vi "FGV_DOCK_records_display.vi"(7 "options":T1, 8 "error_in":errorcluster, 11 "input":variant) -> (0 "error_out":errorcluster, 3 "output":variant)   [LabVIEW 2019]
uses:
  FGV_DOCK_records_display.ctl
  DOCK_references.ctl
  DOCK_all_info.ctl
  DOCK_reference_data.ctl
  MAIN/DOCK_header_data_display.ctl
  DOCK_gear_statuses.ctl
  _misc/AULocalize/SubVIs/Get Localized Phrase Compact Interface 0D.vi
  _misc/AULocalize/SubVIs/Get Localized Phrase Compact Interface 1D.vi
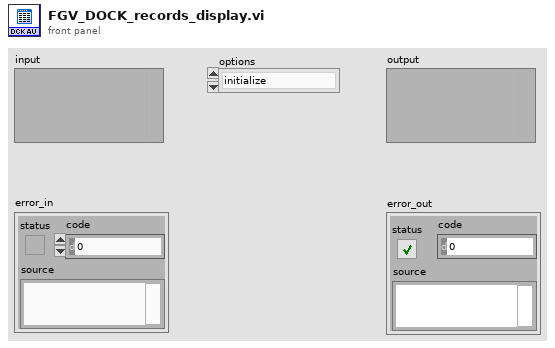
[diagram p1: front panel]
types:
  T1 = typedef "FGV_DOCK_records_display.ctl" = enum16{"initialize", "set_reference_data", "set_serial", "set_header", "set_operations", "set_results", "set_batches", "get_reference_data", "get_part_number_ref", "get_serial", "get_batch_code", "get_gear_ID", "get_operation_IDs", "toggle_results", "show_all_results", "hide_all_results", "display", "clear"}
  T2 = typedef "DOCK_all_info.ctl" = cluster{"reference_data":T3, "serial":string, "DOCK_header":T4, "operations":string[][], "operation_statuses":T5[], "results":string[][], "result_statuses":T5[], "batches":string[][], "batch_statuses":T5[], "DOCK_references":T6}
  T3 = typedef "DOCK_reference_data.ctl" = cluster{"part_number_ref":string, "part_name_ref":string, "PSW_ref":string, "AUSS_ref":string}
  T4 = typedef "DOCK_header_data_display.ctl" = cluster{"ID":string, "creation_time":string, "last_station":string, "last_status":string, "pinion_serial":string, "batch_code":string}
  T5 = typedef "DOCK_GEAR_statuses.ctl" = enum16{"OP_OK_hide", "OP_OK_show", "OP_NOK_hide", "OP_NOK_show", "OP_interrupted_hide", "OP_interrupted_show", "OP_in_operation_hide", "OP_in_operation_show", "OP_unexpected_hide", "OP_unexpected_show", "RE_REAL_OK", "RE_REAL_NOK", "RE_STRING", "RE_sub_header", "RE_no_data", "RE_unexpected", "BA_sub_header", "BA_data", "BA_no_data"}
  T6 = typedef "DOCK_references.ctl" = cluster{"front_panel_reference":refnum<vi>, "SQL_listbox_reference":refnum<vi>, "DOCK_header_data_display":refnum<vi>}
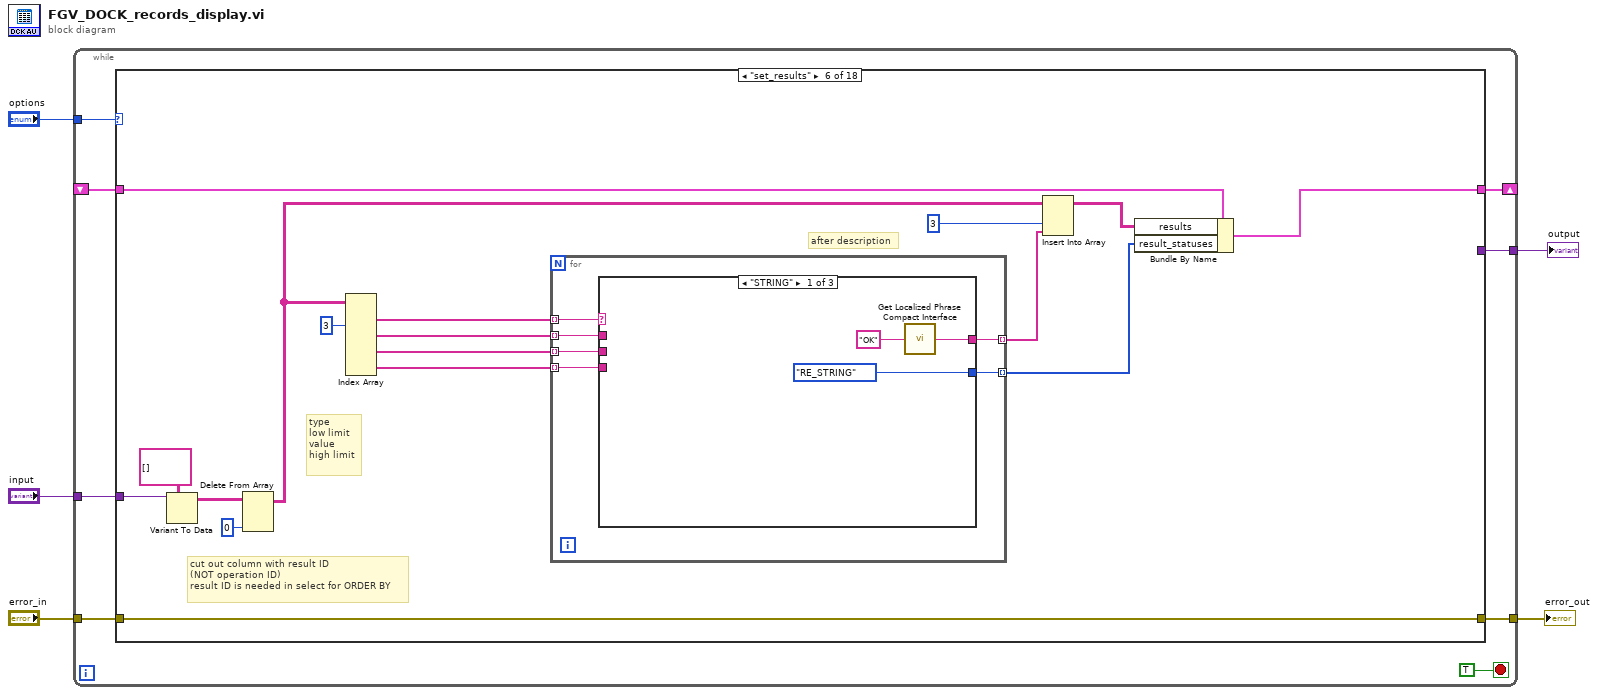
[diagram p0: block diagram]
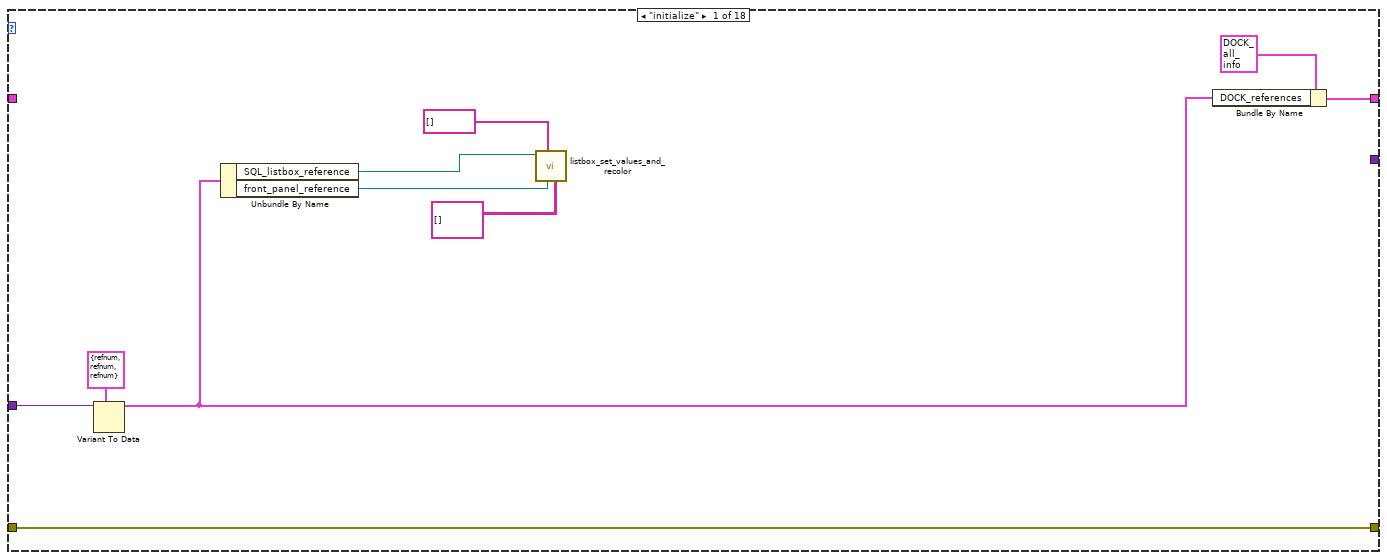
[diagram p2: hidden frame]
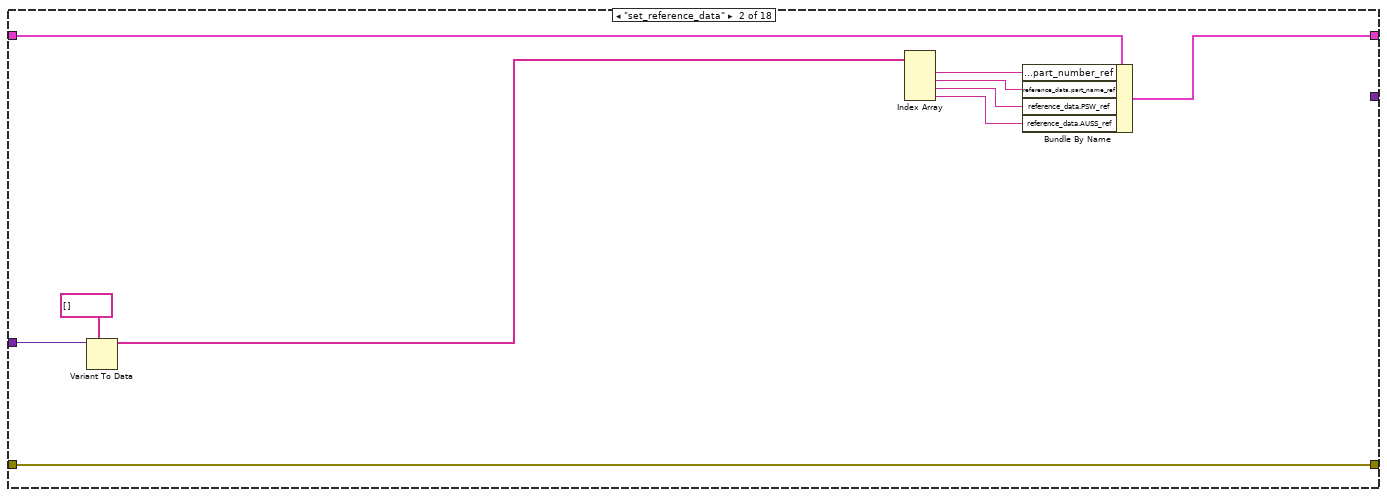
[diagram p3: hidden frame]
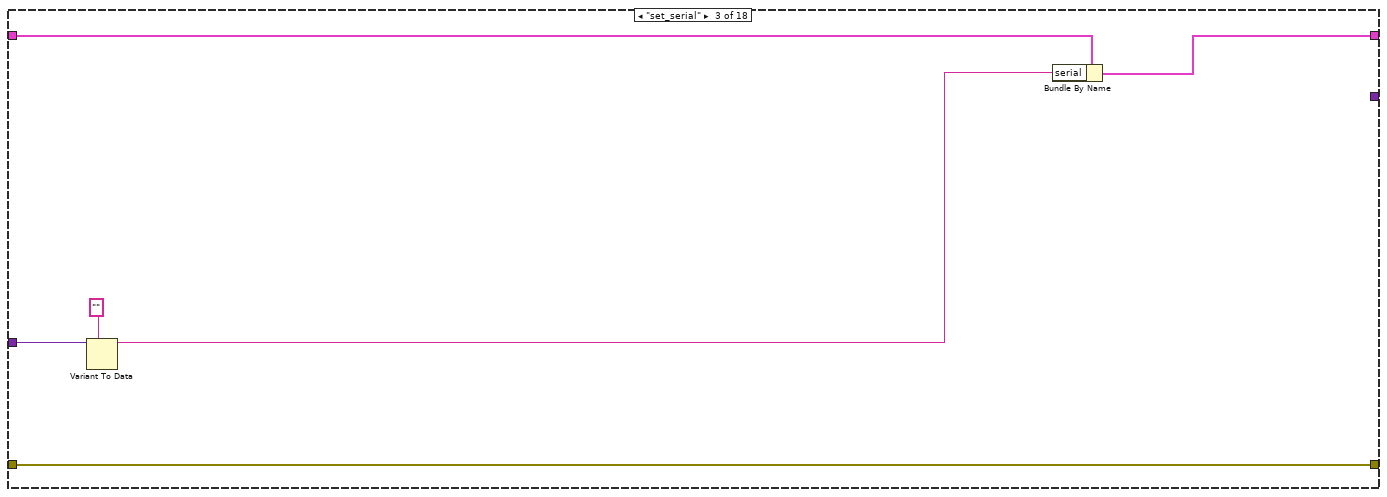
[diagram p4: hidden frame]
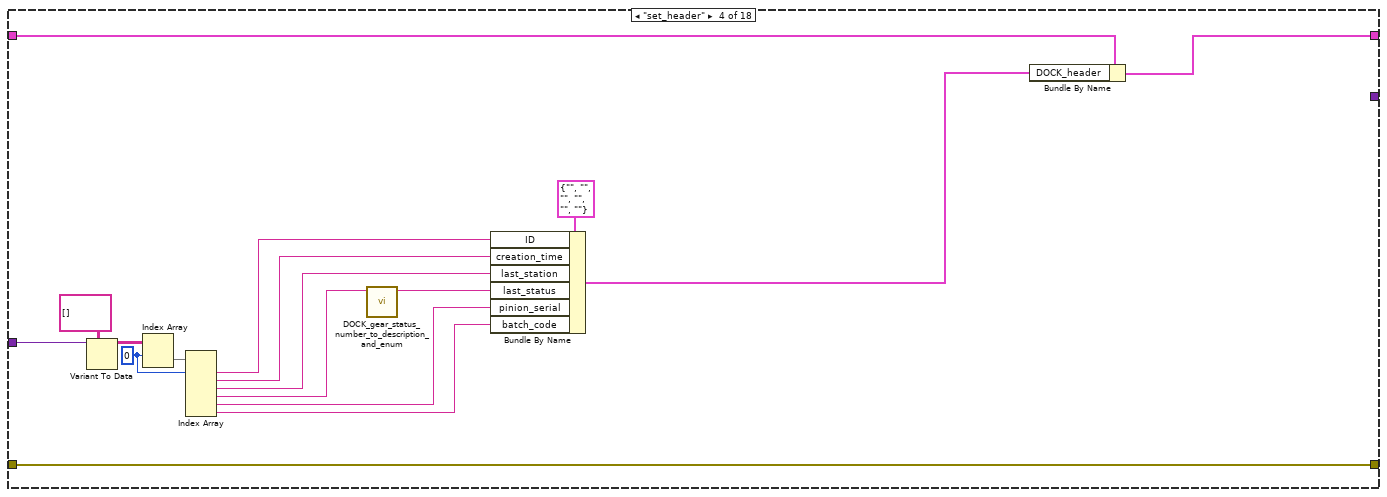
[diagram p5: hidden frame]
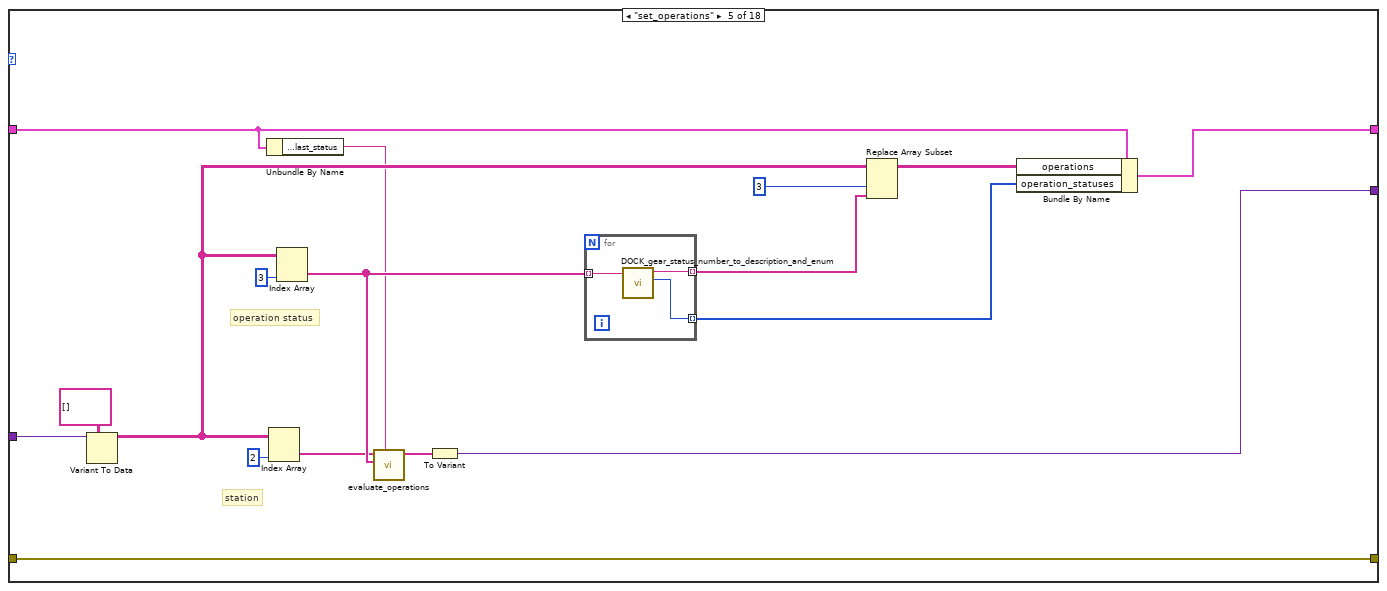
[diagram p6: hidden frame]
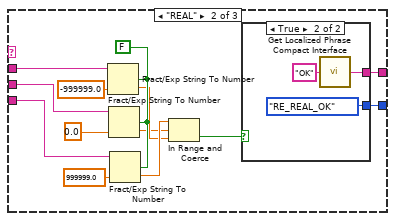
[diagram p7: hidden frame]
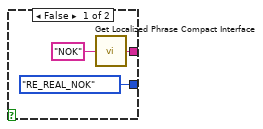
[diagram p8: hidden frame]
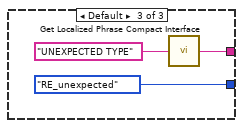
[diagram p9: hidden frame]
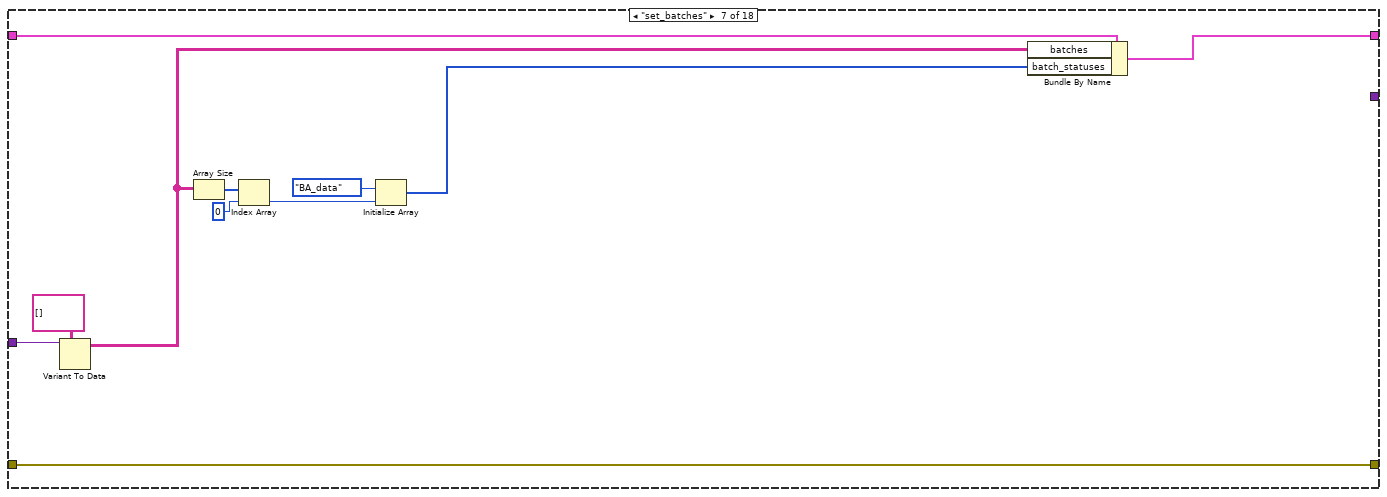
[diagram p10: hidden frame]
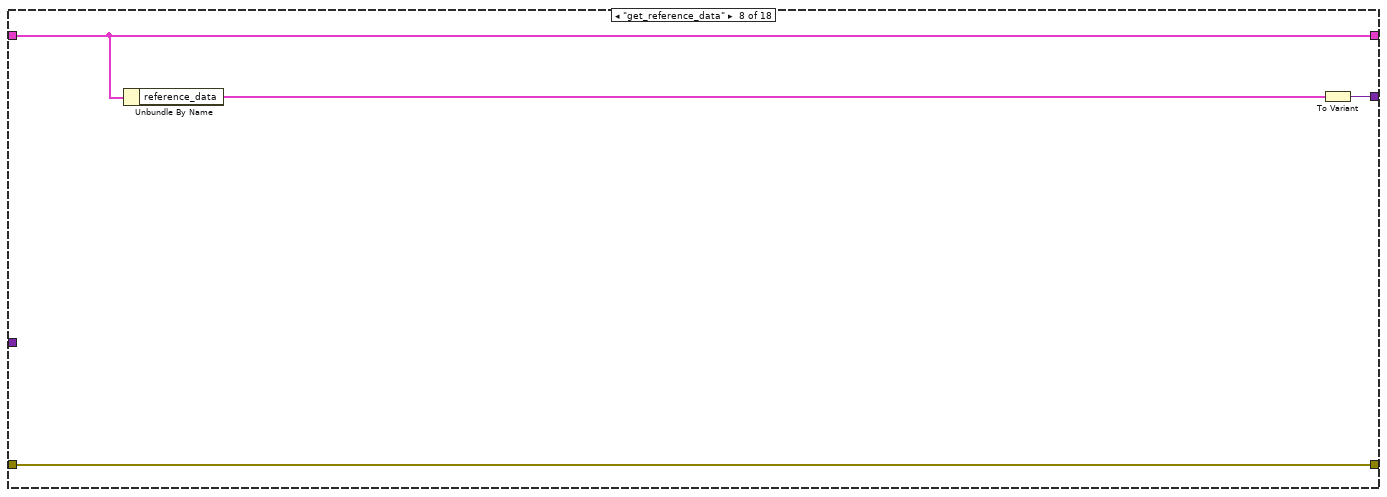
[diagram p11: hidden frame]
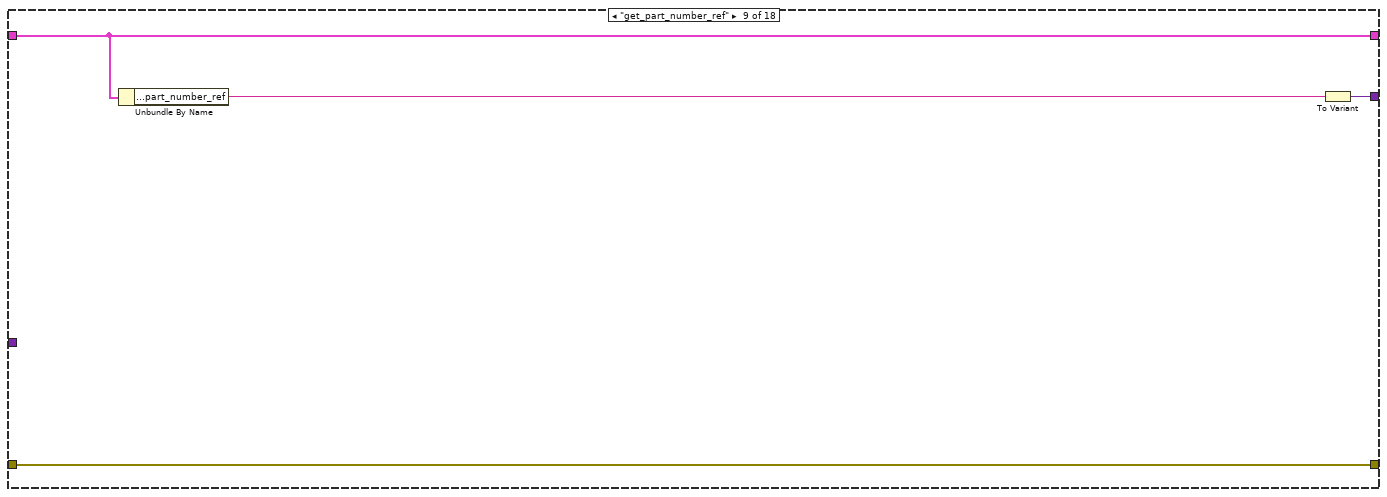
[diagram p12: hidden frame]
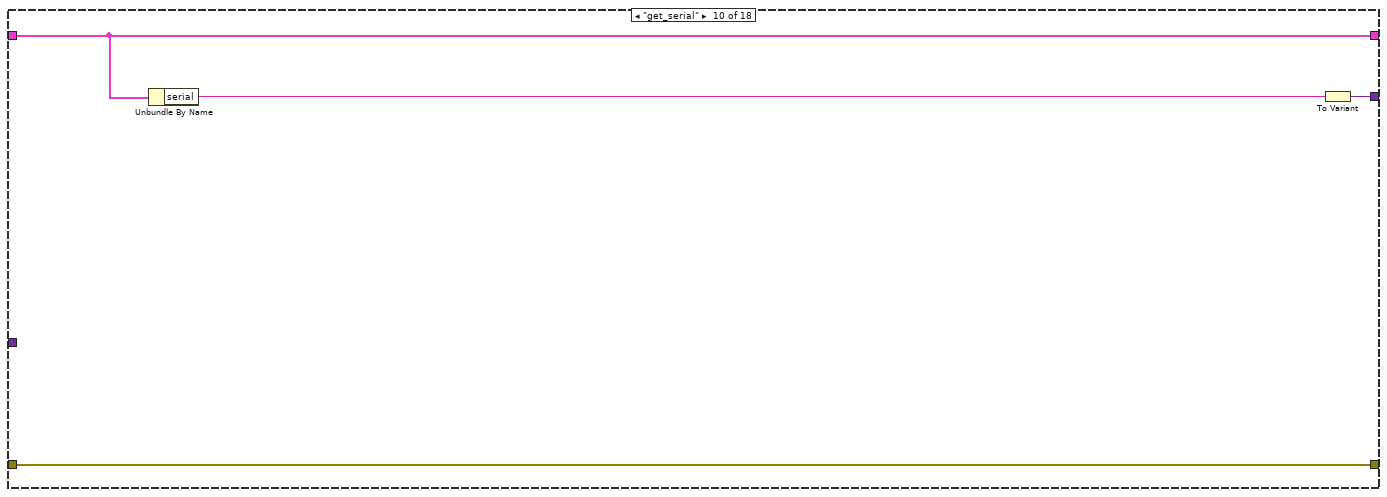
[diagram p13: hidden frame]
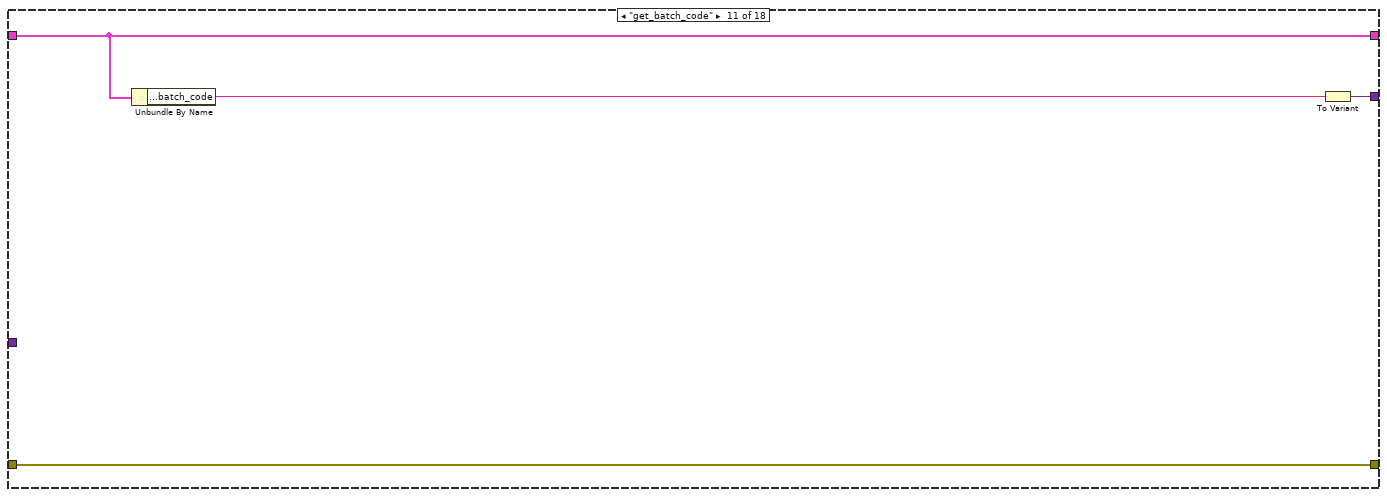
[diagram p14: hidden frame]
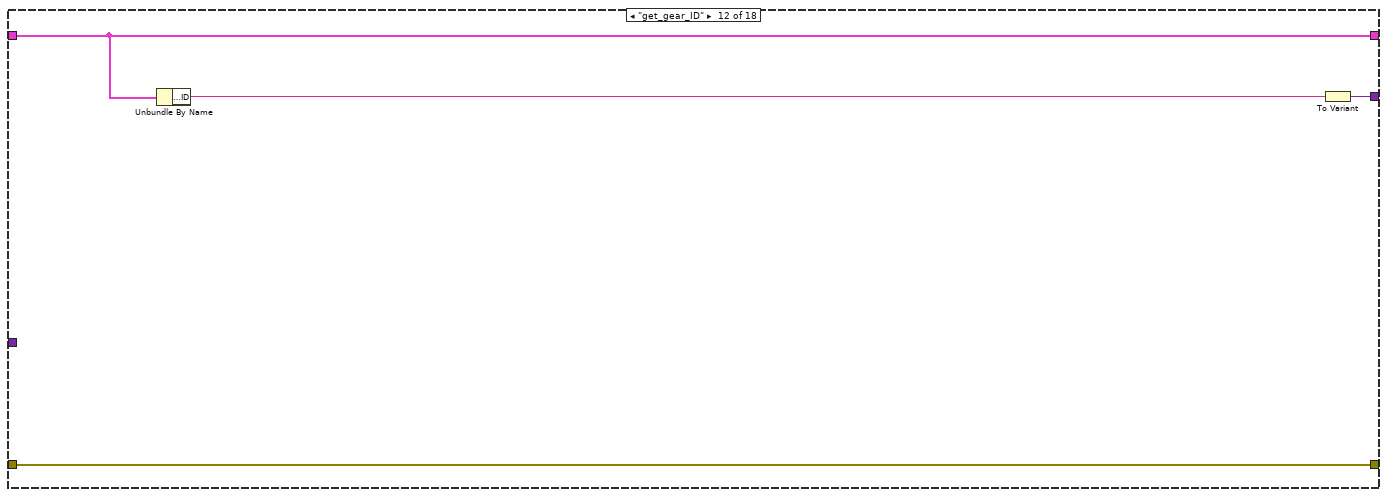
[diagram p15: hidden frame]
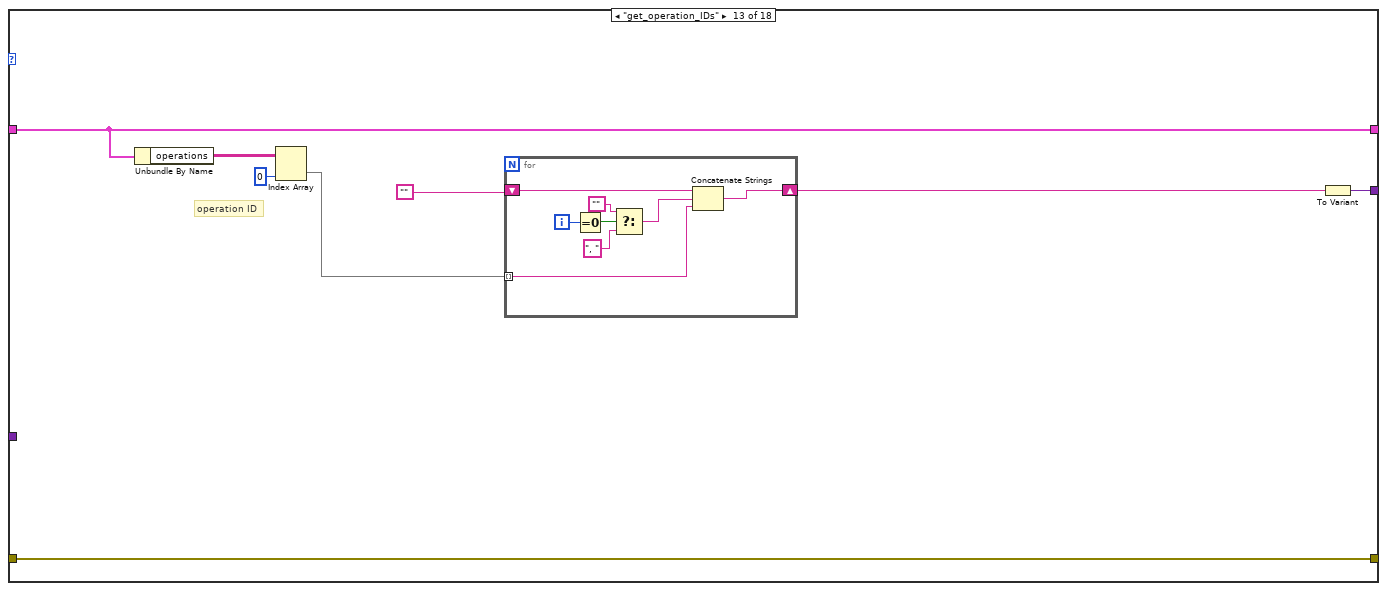
[diagram p16: hidden frame]
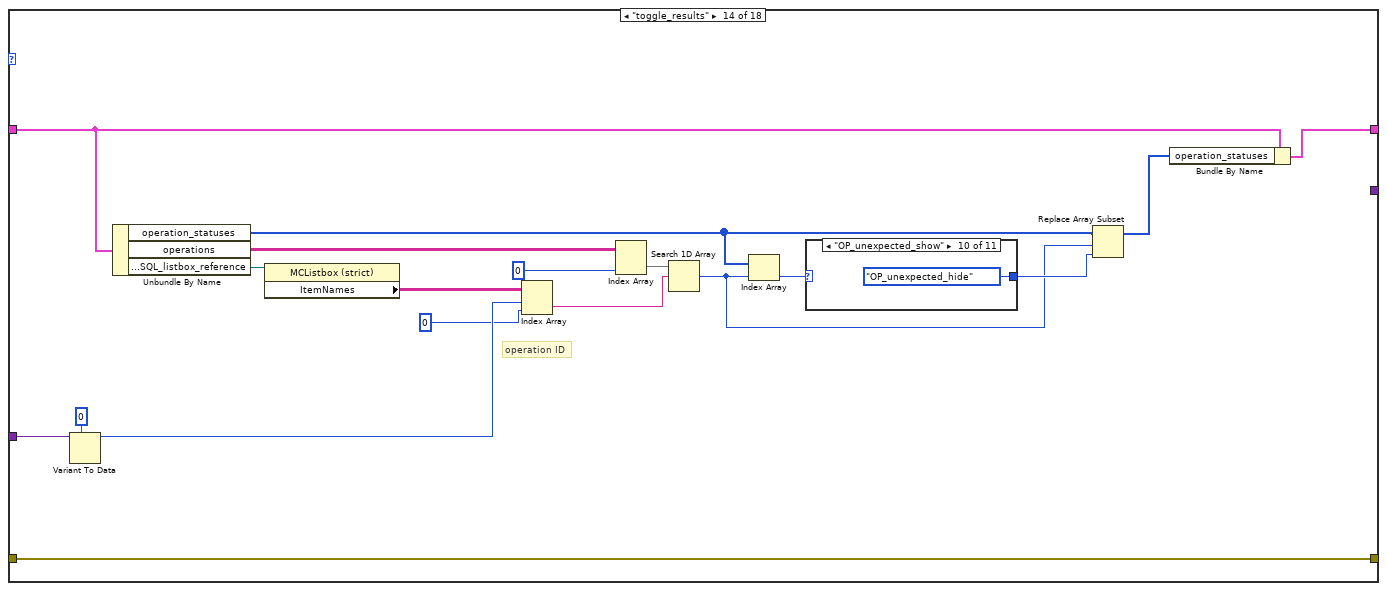
[diagram p17: hidden frame]
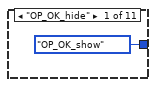
[diagram p18: hidden frame]
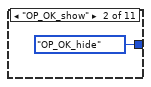
[diagram p19: hidden frame]
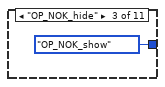
[diagram p20: hidden frame]
diagram:
  n1 = while {
    tunnel: "options" -> [w12]
    tunnel: [w11] -> w5
    tunnel: "error_in" -> [w10]
    shift-right: [w9] -> _
    shift-left: _ -> [w8]
    tunnel: "input" -> [w7]
    tunnel: [w6] -> w1
    stop <- TRUE stop-if-true
    n2 = case shown="\"set_results\"" w12 {
      tunnel: [w23 w33 w39 w56 w73 w93 w135 w139 w143 w147 w151 w155 w163 w189 w205 w218 w232 w244] -> w11
      tunnel: w10 -> [w23 w33 w39 w56 w73 w93 w135 w139 w143 w147 w151 w155 w163 w189 w205 w218 w232 w244]
      tunnel: [w15 w32 w38 w55 w72 w92 w134 w137 w141 w145 w149 w153 w161 w173 w203 w216 w228 w237] -> w9
      tunnel: w8 -> [_ w30 w36 w53 w58 w90 w132 w137 w141 w145 w149 w153 w161 w174 w204 w217 w228 w241]
      tunnel: w7 -> [w19 w31 w37 w54 w71 w91 w133 _ _ _ _ _ _ w187 _ _ _ _]
      tunnel: [_ _ _ _ w59 _ _ w138 w142 w146 w150 w154 w162 _ _ _ _ _] -> w6
      frame "initialize" {
        n3 = Variant To Data(type=T6 {"front_panel_reference"=refnum, "SQL_listbox_reference"=refnum, "DOCK_header_data_display"=refnum} ("REWORK_references"), Variant=w19) -> (data=w16:T6)  [unwired: 1 in, 1 out]
        n4 = Unbundle By Name(w16) -> ("SQL_listbox_reference"=w17:refnum<vi>, "front_panel_reference"=w18:refnum<vi>)
        n5 = call "listbox_set_values_and_recolor.vi"("item_names"=string[][] [], "front_panel_reference"=w18, "column_names"=string[] [], "multicolumn_listbox_reference_in"=w17) -> ()  [unwired: 6 in, 2 out]
        n6 = Bundle By Name(cluster=T2 {"reference_data"={"part_number_ref"="", "part_name_ref"="", "PSW_ref"="", "AUSS_ref"=""}, "serial"="", "DOCK_header"={"ID"="", "creation_time"="", "last_station"="", "last_status"="", "pinion_serial"="", "batch_code"=""}, "operations"=[], "operation_statuses"=[], "results"=[], "result_statuses"=[], "batches"=[], "batch_statuses"=[], "DOCK_references"={"front_panel_reference"=refnum, "SQL_listbox_reference"=refnum, "DOCK_header_data_display"=refnum}} ("REPORT_all_info"), "DOCK_references"=w16) -> (w15:T2)
      }
      frame "set_reference_data" {
        n7 = Variant To Data(type=string[] [], Variant=w31) -> (data=w28:string[])  [unwired: 1 in, 1 out]
        n8 = Index Array(array=w28) -> (element #1=w27:string, element #2=w26:string, element #3=w25:string, element #4=w24:string)  [unwired: 4 in]
        n9 = Bundle By Name(cluster=w30, "reference_data.part_number_ref"=w27, "reference_data.part_name_ref"=w26, "reference_data.PSW_ref"=w25, "reference_data.AUSS_ref"=w24) -> (w32:T2)
      }
      frame "set_serial" {
        n10 = Variant To Data(type="", Variant=w37) -> (data=w34:string)  [unwired: 1 in, 1 out]
        n11 = Bundle By Name(cluster=w36, "serial"=w34) -> (w38:T2)
      }
      frame "set_header" {
        w47 = 0 ("index (row)")
        n12 = Variant To Data(type=string[][] [], Variant=w54) -> (data=w49:string[][])  [unwired: 1 in, 1 out]
        n13 = Index Array(array=w49, index (row)=w47) -> (element=w48:string[])  [unwired: 1 in]
        n14 = Index Array(array=w48, index #1=w47) -> (element #1=w45:string, element #2=w46:string, element #3=w44:string, element #4=w42:string, element #5=w43:string, element #6=w40:string)  [unwired: 5 in]
        n15 = call "DOCK_gear_status_number_to_description_and_enum.vi"("status_nmb"=w42) -> ("status_description"=w41:string)  [unwired: 9 in, 1 out]
        n16 = Bundle By Name(cluster=T4 {"ID"="", "creation_time"="", "last_station"="", "last_status"="", "pinion_serial"="", "batch_code"=""} ("REPORT_GEAR_header_data_display"), "ID"=w45, "creation_time"=w46, "last_station"=w44, "last_status"=w41, "pinion_serial"=w43, "batch_code"=w40) -> (w50:T4)
        n17 = Bundle By Name(cluster=w53, "DOCK_header"=w50) -> (w55:T2)
      }
      frame "set_operations" {
        # "station"
        # "operation status"
        n18 = Variant To Data(type=string[][] [], Variant=w71) -> (data=w63:string[][])  [unwired: 1 in, 1 out]
        n19 = Unbundle By Name(w58) -> ("DOCK_header.last_status"=w57:string)
        n20 = Index Array(array=w63, index (col)=2 ("disabled index (col)")) -> (element=w61:string[])  [unwired: 1 in]
        n21 = Index Array(array=w63, index (col)=3 ("disabled index (col)")) -> (element=w62:string[])  [unwired: 1 in]
        n22 = call "evaluate_operations.vi"("last_status"=w57, "operation_statuses"=w62, "stations"=w61) -> ("NOK_stations"=w60:string[])  [unwired: 8 in]
        n23 = To Variant(anything=w60) -> (Variant=w59:variant)
        n24 = for {
          tunnel: w62 -> [w76] mode=indexing
          tunnel: [w75] -> w68 mode=indexing
          tunnel: [w74] -> w65 mode=indexing
          n25 = call "DOCK_gear_status_number_to_description_and_enum.vi"("status_nmb"=w76) -> ("status_enum"=w75:T5, "status_description"=w74:string)  [unwired: 9 in]
        }
        n26 = Replace Array Subset(array=w63, new element=w65, index (col)=3 ("disabled index (col)")) -> (w66:string[][])  [unwired: 1 in]
        n27 = Bundle By Name(cluster=w58, "operations"=w66, "operation_statuses"=w68) -> (w72:T2)
      }
      frame "set_results" {
        # "after description"
        # "cut out column with result ID\n(NOT operation ID)\nresult ID is needed in select for ORDER BY"
        # "type\nlow limit\nvalue\nhigh limit"
        n28 = Variant To Data(type=string[][] [], Variant=w91) -> (data=w80:string[][])  [unwired: 1 in, 1 out]
        n29 = Delete From Array(array=w80, index (col)=0 ("disabled index (col)")) -> (array with subset deleted=w79:string[][])  [unwired: 2 in, 1 out]
        n30 = Index Array(array=w79, index (col) #1=3 ("disabled index (col)")) -> (element #1=w83:string[], element #2=w88:string[], element #3=w86:string[], element #4=w85:string[])  [unwired: 7 in]
        n31 = for {
          tunnel: w88 -> [w96] mode=indexing
          tunnel: [w99] -> w87 mode=indexing
          tunnel: [w98] -> w81 mode=indexing
          tunnel: w86 -> [w95] mode=indexing
          tunnel: w85 -> [w94] mode=indexing
          tunnel: w83 -> [w97] mode=indexing
          n32 = case shown="\"STRING\"" w97 {
            tunnel: [DOCK_GEAR_statuses."RE_STRING" ("REPORT_GEAR_statuses") w115 DOCK_GEAR_statuses."RE_unexpected" ("REPORT_GEAR_statuses")] -> w99
            tunnel: [w100 w114 w122] -> w98
            tunnel: w96 -> [_ w113 _]
            tunnel: w95 -> [_ w111 _]
            tunnel: w94 -> [_ w110 _]
            frame "STRING" {
              n33 = call-poly "Get Localized Phrase Compact Interface.vi"("Key"="OK") -> ("Translated Phrase"=w100:string)
            }
            frame "REAL" {
              w112 = FALSE ("use system decimal point (T)")
              n34 = Fract/Exp String To Number(use system decimal point (T)=w112, string=w113, default (0 dbl)=sgl -999999.0 ("default (0 DBL)")) -> (number=w108:sgl)  [unwired: 1 in, 1 out]
              n35 = Fract/Exp String To Number(use system decimal point (T)=w112, string=w111, default (0 dbl)=sgl 0.0 ("default (0 DBL)")) -> (number=w107:sgl)  [unwired: 1 in, 1 out]
              n36 = Fract/Exp String To Number(use system decimal point (T)=w112, string=w110, default (0 dbl)=sgl 999999.0 ("default (0 DBL)")) -> (number=w109:sgl)  [unwired: 1 in, 1 out]
              n37 = In Range and Coerce(upper limit=w109, x=w107, lower limit=w108) -> (In Range?=w106:bool)  [unwired: 1 out]
              n38 = case shown="True" w106 {
                tunnel: [DOCK_GEAR_statuses."RE_REAL_NOK" ("REPORT_GEAR_statuses") DOCK_GEAR_statuses."RE_REAL_OK" ("REPORT_GEAR_statuses")] -> w115
                tunnel: [w116 w119] -> w114
                frame False {
                  n39 = call-poly "Get Localized Phrase Compact Interface.vi"("Key"="NOK") -> ("Translated Phrase"=w116:string)
                }
                frame True {
                  n40 = call-poly "Get Localized Phrase Compact Interface.vi"("Key"="OK") -> ("Translated Phrase"=w119:string)
                }
              }
            }
            frame Default {
              n41 = call-poly "Get Localized Phrase Compact Interface.vi"("Key"="UNEXPECTED TYPE") -> ("Translated Phrase"=w122:string)
            }
          }
        }
        n42 = Insert Into Array(array=w79, index (col)=3 ("disabled index (col)"), new element=w81) -> (w82:string[][])  [unwired: 1 in]
        n43 = Bundle By Name(cluster=w90, "results"=w82, "result_statuses"=w87) -> (w92:T2)
      }
      frame "set_batches" {
        n44 = Variant To Data(type=string[][] [], Variant=w133) -> (data=w129:string[][])  [unwired: 1 in, 1 out]
        n45 = Array Size(array=w129) -> (size(s)=w128:i32[])
        n46 = Index Array(array=w128, index=0) -> (element=w126:i32)
        n47 = Initialize Array(DOCK_GEAR_statuses."BA_data" ("REPORT_GEAR_statuses"), w126) -> (w125:T5[])
        n48 = Bundle By Name(cluster=w132, "batches"=w129, "batch_statuses"=w125) -> (w134:T2)
      }
      frame "get_reference_data" {
        n49 = Unbundle By Name(w137) -> ("reference_data"=w136:T3)
        n50 = To Variant(anything=w136) -> (Variant=w138:variant)
      }
      frame "get_part_number_ref" {
        n51 = Unbundle By Name(w141) -> ("reference_data.part_number_ref"=w140:string)
        n52 = To Variant(anything=w140) -> (Variant=w142:variant)
      }
      frame "get_serial" {
        n53 = Unbundle By Name(w145) -> ("serial"=w144:string)
        n54 = To Variant(anything=w144) -> (Variant=w146:variant)
      }
      frame "get_batch_code" {
        n55 = Unbundle By Name(w149) -> ("DOCK_header.batch_code"=w148:string)
        n56 = To Variant(anything=w148) -> (Variant=w150:variant)
      }
      frame "get_gear_ID" {
        n57 = Unbundle By Name(w153) -> ("DOCK_header.ID"=w152:string)
        n58 = To Variant(anything=w152) -> (Variant=w154:variant)
      }
      frame "get_operation_IDs" {
        # "operation ID"
        n59 = Unbundle By Name(w161) -> ("operations"=w160:string[][])
        n60 = Index Array(array=w160, index (col)=0 ("disabled index (col)")) -> (element=w158:string[])  [unwired: 1 in]
        n61 = for {
          tunnel: w158 -> [w164] mode=indexing
          shift-right: [w167] -> w156
          shift-left: "" -> [w166]
          i -> [w168]
          n62 = Equal To 0?(x=w168) -> (x = 0?=w169:bool)
          n63 = Select(t="", s=w169, f=", ") -> (s? t:f=w165:string)
          n64 = Concatenate Strings(w166, w165, w164) -> (w167:string)
        }
        n65 = To Variant(anything=w156) -> (Variant=w162:variant)
      }
      frame "toggle_results" {
        # "operation ID"
        n66 = Variant To Data(type=0 ("Row"), Variant=w187) -> (data=w184:i32)  [unwired: 1 in, 1 out]
        n67 = Unbundle By Name(w174) -> ("operation_statuses"=w177:T5[], "operations"=w182:string[][], "DOCK_references.SQL_listbox_reference"=w188:refnum<vi>)
        n68 = property class="MCListbox (strict)"(reference=w188) -> ("ItemNames"=w185:string[][])  [unwired: 1 in, 2 out]
        n69 = Index Array(array=w185, index (row)=w184, index (col)=0 ("disabled index (col)")) -> (element=w179:string)
        n70 = Index Array(array=w182, index (col)=0 ("disabled index (col)")) -> (element=w180:string[])  [unwired: 1 in]
        n71 = Search 1D Array(1D array=w180, element=w179) -> (index of element=w175:i32)  [unwired: 1 in]
        n72 = Index Array(array=w177, index=w175) -> (element=w178:T5)
        n73 = case shown="\"OP_unexpected_show\"" w178 {
          selector: w178 -> [_ _ _ _ _ _ _ _ _ _ w200]
          tunnel: [DOCK_GEAR_statuses."OP_OK_show" ("REPORT_GEAR_statuses") DOCK_GEAR_statuses."OP_OK_hide" ("REPORT_GEAR_statuses") DOCK_GEAR_statuses."OP_NOK_show" ("REPORT_GEAR_statuses") DOCK_GEAR_statuses."OP_NOK_hide" ("REPORT_GEAR_statuses") DOCK_GEAR_statuses."OP_interrupted_show" ("REPORT_GEAR_statuses") DOCK_GEAR_statuses."OP_interrupted_hide" ("REPORT_GEAR_statuses") DOCK_GEAR_statuses."OP_in_operation_show" ("REPORT_GEAR_statuses") DOCK_GEAR_statuses."OP_in_operation_hide" ("REPORT_GEAR_statuses") DOCK_GEAR_statuses."OP_unexpected_show" ("REPORT_GEAR_statuses") DOCK_GEAR_statuses."OP_unexpected_hide" ("REPORT_GEAR_statuses") w200] -> w176
          frame "OP_OK_hide" {
          }
          frame "OP_OK_show" {
          }
          frame "OP_NOK_hide" {
          }
          frame "OP_NOK_show" {
          }
          frame "OP_interrupted_hide" {
          }
          frame "OP_interrupted_show" {
          }
          frame "OP_in_operation_hide" {
          }
          frame "OP_in_operation_show" {
          }
          frame "OP_unexpected_hide" {
          }
          frame "OP_unexpected_show" {
          }
          frame Default {
          }
        }
        n74 = Replace Array Subset(array=w177, new element=w176, index=w175) -> (w172:T5[])
        n75 = Bundle By Name(cluster=w174, "operation_statuses"=w172) -> (w173:T2)
      }
      frame "show_all_results" {
        n76 = Unbundle By Name(w204) -> ("operation_statuses"=w202:T5[])
        n77 = for {
          tunnel: w202 -> [w207] mode=indexing
          tunnel: [w206] -> w201 mode=indexing
          n78 = case shown="Default" w207 {
            selector: w207 -> [_ _ _ _ _ w213]
            tunnel: [DOCK_GEAR_statuses."OP_OK_show" ("REPORT_GEAR_statuses") DOCK_GEAR_statuses."OP_NOK_show" ("REPORT_GEAR_statuses") DOCK_GEAR_statuses."OP_interrupted_show" ("REPORT_GEAR_statuses") DOCK_GEAR_statuses."OP_in_operation_show" ("REPORT_GEAR_statuses") DOCK_GEAR_statuses."OP_unexpected_show" ("REPORT_GEAR_statuses") w213] -> w206
            frame "OP_OK_hide" {
            }
            frame "OP_NOK_hide" {
            }
            frame "OP_interrupted_hide" {
            }
            frame "OP_in_operation_hide" {
            }
            frame "OP_unexpected_hide" {
            }
            frame Default {
            }
          }
        }
        n79 = Bundle By Name(cluster=w204, "operation_statuses"=w201) -> (w203:T2)
      }
      frame "hide_all_results" {
        n80 = Unbundle By Name(w217) -> ("operation_statuses"=w215:T5[])
        n81 = for {
          tunnel: w215 -> [w219] mode=indexing
          tunnel: [w220] -> w214 mode=indexing
          n82 = case shown="\"OP_unexpected_show\"" w219 {
            selector: w219 -> [_ _ _ _ _ w226]
            tunnel: [DOCK_GEAR_statuses."OP_OK_hide" ("REPORT_GEAR_statuses") DOCK_GEAR_statuses."OP_NOK_hide" ("REPORT_GEAR_statuses") DOCK_GEAR_statuses."OP_interrupted_hide" ("REPORT_GEAR_statuses") DOCK_GEAR_statuses."OP_in_operation_hide" ("REPORT_GEAR_statuses") DOCK_GEAR_statuses."OP_unexpected_hide" ("REPORT_GEAR_statuses") w226] -> w220
            frame "OP_OK_show" {
            }
            frame "OP_NOK_show" {
            }
            frame "OP_interrupted_show" {
            }
            frame "OP_in_operation_show" {
            }
            frame "OP_unexpected_show" {
            }
            frame Default {
            }
          }
        }
        n83 = Bundle By Name(cluster=w217, "operation_statuses"=w214) -> (w216:T2)
      }
      frame "display" {
        n84 = Unbundle By Name(w228) -> ("DOCK_references.DOCK_header_data_display"=w231:refnum<vi>, "DOCK_header"=w230:T4)
        n85 = call-poly "Get Localized Phrase Compact Interface.vi"("Key"=string[] ["ID", "Time", "OP", "Status", "Operator"] ("column_names")) -> ("Translated Phrase"=w227:string[])
        n86 = call "DOCK_listbox_set_values_and_recolor.vi"("column_names"=w227, "REPORT_all_info"=w228) -> ()  [unwired: 9 in, 1 out]
        n87 = property class="Clust (strict)"(reference=w231, "Value"=w230) -> ()  [unwired: 1 in, 2 out]
      }
      frame "clear" {
        n88 = Unbundle By Name(w241) -> ("reference_data"=w233:T3, "DOCK_references"=w238:T6, "DOCK_references.SQL_listbox_reference"=w240:refnum<vi>, "DOCK_references.front_panel_reference"=w239:refnum<vi>, "DOCK_references.DOCK_header_data_display"=w235:refnum<vi>)
        n89 = property class="Clust (strict)"(reference=w235, "Value"=T4 {"ID"="", "creation_time"="", "last_station"="", "last_status"="", "pinion_serial"="", "batch_code"=""}) -> ()  [unwired: 1 in, 2 out]
        n90 = call "listbox_set_values_and_recolor.vi"("item_names"=string[][] [], "front_panel_reference"=w239, "column_names"=string[] [], "multicolumn_listbox_reference_in"=w240) -> ()  [unwired: 6 in, 2 out]
        n91 = Bundle By Name(cluster=T2 {"reference_data"={"part_number_ref"="", "part_name_ref"="", "PSW_ref"="", "AUSS_ref"=""}, "serial"="", "DOCK_header"={"ID"="", "creation_time"="", "last_station"="", "last_status"="", "pinion_serial"="", "batch_code"=""}, "operations"=[], "operation_statuses"=[], "results"=[], "result_statuses"=[], "batches"=[], "batch_statuses"=[], "DOCK_references"={"front_panel_reference"=refnum, "SQL_listbox_reference"=refnum, "DOCK_header_data_display"=refnum}} ("REPORT_all_info"), "reference_data"=w233, "DOCK_references"=w238) -> (w237:T2)
      }
    }
  }
  "error_out" <- w5
  "output" <- w1
